vi "rtlsdr_read_to_queue.vi"(7 "ref in":refnum<k5>, 8 "error in (no error)":errorcluster, 9 "buffer size":i32=1024, 10 "iq queue in":T1) -> (0 "error out":errorcluster, 2 "iq queue out":T1, 5 "ref out":refnum<k5>)   [LabVIEW 2011]
uses:
  iq_queue_typedef_out.ctl
panel:
  # "Outputs:"
  # "Inputs:"
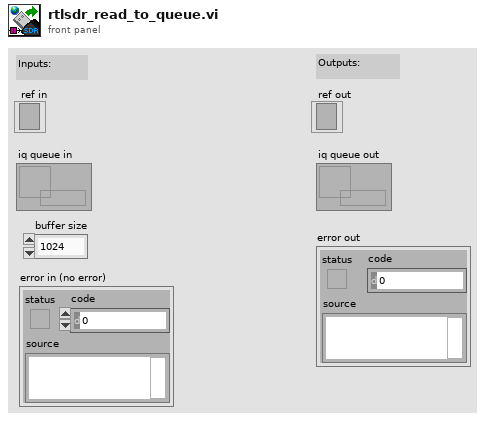
[diagram p1: front panel]
types:
  T1 = typedef "iq_queue_typedef_out.ctl" = refnum<queue>
  T2 = enum16{"Standard", "Buffered", "CRLF", "Immediate"}
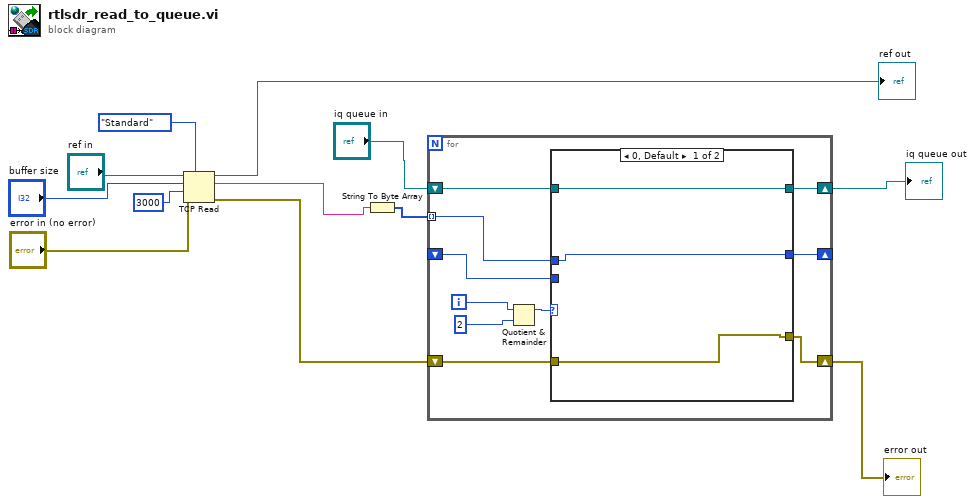
[diagram p0: block diagram]
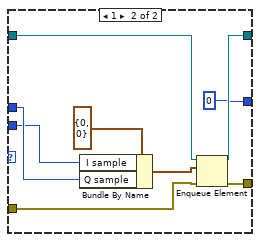
[diagram p2: hidden frame]
diagram:
  n1 = TCP Read(connection ID="ref in", bytes to read="buffer size", error in (no error)="error in (no error)", 7:T2."Standard" ("mode (standard)"), 9:3000 ("timeout ms (25000)")) -> (connection ID out=→"ref out":refnum<k5>, data out=w6:string, error out=w1:errorcluster)
  n2 = String To Byte Array(string=w6) -> (unsigned byte array=w5:u8[])
  n3 = for {
    tunnel: w5 -> [w19] mode=indexing
    shift-right: [w18] -> _
    shift-left: _ -> [w17]
    shift-right: [w15] -> w3
    shift-left: "iq queue in" -> [w16]
    shift-right: [w14] -> w2
    shift-left: w1 -> [w13]
    i -> [w22]
    n4 = Quotient & Remainder(x=w22, y=2) -> (x-y*floor(x/y)=w20:i32)  [unwired: 1 out]
    n5 = case shown="0, Default" w20 {
      tunnel: w19 -> [w25 w33]
      tunnel: [w25 u8 0] -> w18
      tunnel: w17 -> [_ w32]
      tunnel: w16 -> [w23 w31]
      tunnel: [w23 w30] -> w15
      tunnel: w13 -> [w24 w28]
      tunnel: [w24 w27] -> w14
      frame 0, Default {
      }
      frame 1 {
        n6 = Bundle By Name(cluster=cluster{"I sample":u8, "Q sample":u8} {"I sample"=0, "Q sample"=0} ("I/Q sample cluster"), "I sample"=w32, "Q sample"=w33) -> (w29:cluster{"I sample":u8, "Q sample":u8})
        n7 = Enqueue Element(queue=w31, element=w29, error in (no error)=w28) -> (queue out=w30:T1, error out=w27:errorcluster)  [unwired: 1 in, 1 out]
      }
    }
  }
  "error out" <- w2
  "iq queue out" <- w3
